vi "Second tens.vi"(8 "error in (no error)":errorcluster, 10 "Time Stamp":timestamp) -> (0 "error out":errorcluster, 2 "Time Stamp 2":timestamp, 3 "Second Ones":bool[](array[boolean]))   [LabVIEW 2014]
uses:
  <vilib>/myRIO/Instrument Drivers/Onboard IO/DIO/typedefs/DIO Reference.ctl
  <vilib>/myRIO/Common/Instrument Driver Framework/Utilities/typedefs/myRIO Generic Hardware Reference.ctl
  <vilib>/myRIO/Common/Instrument Driver Framework/Utilities/typedefs/Hardware Version Enum.ctl
  <vilib>/myRIO/Common/Instrument Driver Framework/Utilities/typedefs/myRIO v1.0 Reference.ctl
  <vilib>/myRIO/Common/Instrument Driver Framework/Utilities/typedefs/Generic FPGA Reference.ctl
  <vilib>/myRIO/Common/Instrument Driver Framework/myRIO v1.0/DIO/typedefs/DIO Channels List.ctl
  <vilib>/myRIO/Common/Instrument Driver Framework/myRIO v1.0/DIO/typedefs/DIO Channels Enum.ctl
  <vilib>/userdefined/High Color/nirio_resource_hc.ctl
  <vilib>/myRIO/Common/Instrument Driver Framework/Utilities/vis/Is FPGA Ref Available.vi
  <vilib>/myRIO/Common/Instrument Driver Framework/myRIO v1.0/DIO/vis/myRIO v1.1 Open DIO.vi
  <vilib>/myRIO/Instrument Drivers/Onboard IO/DIO/vis/Write.vi
  <vilib>/myRIO/Common/Instrument Driver Framework/Utilities/vis/Validate Channels.vi
  <vilib>/myRIO/Common/Instrument Driver Framework/myRIO v1.0/DIO/vis/myRIO v1.0 Reserve DIO.vi
  <vilib>/myRIO/Common/Instrument Driver Framework/myRIO v1.0/Resource Manager/vis/myRIO v1.0 Reserve Channel List.vi
  <vilib>/myRIO/Common/Instrument Driver Framework/myRIO v1.0/DIO/vis/myRIO v1.0 Build MUX Configuration DIO.vi
  <vilib>/myRIO/Common/Instrument Driver Framework/myRIO v1.0/Resource Manager/vis/myRIO v1.0 Reserve Channel.vi
  <vilib>/myRIO/Common/Instrument Driver Framework/myRIO v1.0/Resource Manager/vis/myRIO v1.0 Unreserve Channel.vi
  <vilib>/myRIO/Common/Instrument Driver Framework/myRIO v1.0/Resource Manager/vis/myRIO v1.0 Create Configuration List.vi
  <vilib>/myRIO/Common/Instrument Driver Framework/myRIO v1.0/Resource Manager/vis/myRIO v1.0 Build Mutex Name.vi
  <vilib>/Utility/VariantDataType/GetNumericInfo.vi
  <vilib>/Utility/error.llb/Error Cluster From Error Code.vi
  <vilib>/myRIO/Common/Instrument Driver Framework/myRIO v1.0/myRIO v1.1 Open.vi
  <vilib>/myRIO/Common/Instrument Driver Framework/Utilities/vis/IO Manager.vi
  <vilib>/myRIO/Common/Instrument Driver Framework/Utilities/vis/Configuration Manager.vi
  <vilib>/myRIO/Common/Instrument Driver Framework/myRIO v1.0/Resource Manager/vis/myRIO v1.0 Configure IO.vi
  <vilib>/myRIO/Common/Instrument Driver Framework/myRIO v1.0/myRIO v1.0 Close.vi
  <vilib>/myRIO/Common/Instrument Driver Framework/myRIO v1.0/DIO/vis/myRIO v1.0 Write DIO.vi
  <vilib>/myRIO/Express VI/Onboard IO/DO/DO Express VI.xnode
  <vilib>/myRIO/Instrument Drivers/Onboard IO/DIO/vis/myRIO DIO Open.xnode
  <vilib>/myRIO/Instrument Drivers/Onboard IO/DIO/DIO.lvlib
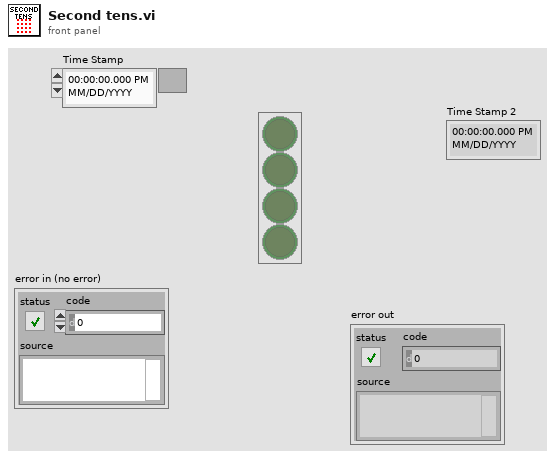
[diagram p1: front panel]
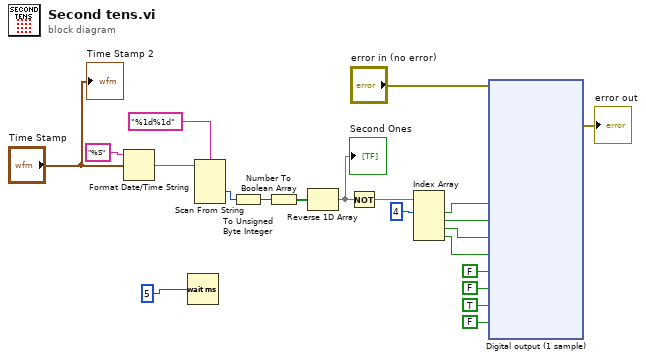
[diagram p0: block diagram]
diagram:
  n1 = Format Date/Time String(time format string (%c)="%S", seconds (now)="Time Stamp") -> (date/time string=w19:string)  [unwired: 1 in]
  n2 = Wait (ms)(milliseconds to wait=u32 5) -> ()  [unwired: 1 out]
  n3 = Scan From String(format string="%1d%1d", input string=w19) -> (output 1=w1:i32)  [unwired: 5 in, 3 out]
  n4 = To Unsigned Byte Integer(number=w1) -> (unsigned 8bit integer=w18:u8)
  n5 = Number To Boolean Array(number=w18) -> (Boolean array=w8:bool[])
  n6 = Reverse 1D Array(array=w8) -> (reversed array=w6:bool[])
  "Second Ones" <- w6
  n7 = Not(x=w6) -> (.not. x?=w7:bool[])
  n8 = Index Array(array=w7, index #1=4 ("index")) -> (element #1=w12:bool, element #2=w11:bool, element #3=w10:bool, element #4=w9:bool)  [unwired: 3 in]
  n9 = xnode "Digital output (1 sample)"("B/DIO0 (Pin 11)"=w12, "B/DIO1 (Pin 13)"=w11, "B/DIO2 (Pin 15)"=w10, "B/DIO3 (Pin 17)"=w9, "B/DIO4 (Pin 19)"=FALSE ("B/DIO7 (Pin 25)"), "B/DIO5 (Pin 21)"=FALSE ("B/DIO7 (Pin 25)"), "B/DIO6 (Pin 23)"=TRUE ("B/DIO7 (Pin 25)"), "B/DIO7 (Pin 25)"=FALSE, "error in (no error)"="error in (no error)") -> ("error out"=→"error out":errorcluster)
  "Time Stamp 2" <- "Time Stamp"
